vi "Create Init File.vi"(8 "error in (no error)":errorcluster caption="entrée d'erreur (pas d'erreur)", 9 "Nom du fichier ini":string, 10 "Répertoire de l'appli":path, 11 "UI Cam Basler in":refnum<class "UI Cam Basler.lvclass">) -> (0 "error out":errorcluster caption="sortie d'erreur", 3 "UI Cam Basler out":refnum<class "UI Cam Basler.lvclass">)   [LabVIEW 2023, in "UI Cam Basler.lvclass"]
uses:
  UI Cam Basler.lvclass
  UI Cam Basler.lvclass/UI Cam Basler.ctl
  83761873-ac89-497a-a2f6-ac3f21e5bc55.vi
  83761873-ac89-497a-a2f6-ac3f21e5bc55.vi/659df739-fa42-474c-bf03-f9ba45f35773.vi
  <vilib>/Utility/file.llb/Is Path and Not Empty.vi
  <vilib>/Utility/libraryn.llb/Librarian Path Location.vi
  <userlib>/_OpenG.lib/file/file.llb/File Exists__ogtk.vi
  <userlib>/_OpenG.lib/file/file.llb/File Exists - Scalar__ogtk.vi
  <userlib>/LV-TOML/lib/Parse TOML String.vi
  <userlib>/LV-TOML/lib/TOML to LabVIEW.vi
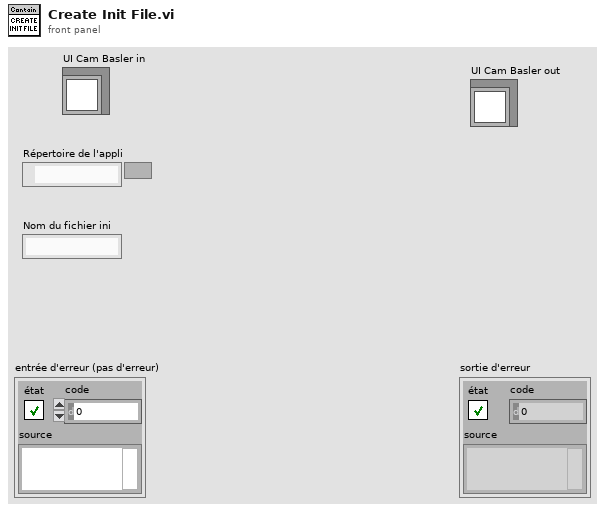
[diagram p1: front panel]
types:
  T1 = enum16{"open", "replace", "create", "open or create", "replace or create", "replace or create with confirmation"}
  T2 = typedef "UI Cam Basler.lvclass/Parsed Data Acquisition.ctl" = cluster{"Config Acquisition":cluster{"Camera name":string, "Gain":dbl, "Shutter(us)":dbl, "ROI":bool, "ROI coor":T3, "Palette":u32, "ModelName":string}}
  T3 = typedef "IMAQ Rectangle" = cluster{"Left":i32, "Top":i32, "Right":i32, "Bottom":i32, "Rotation":dbl}
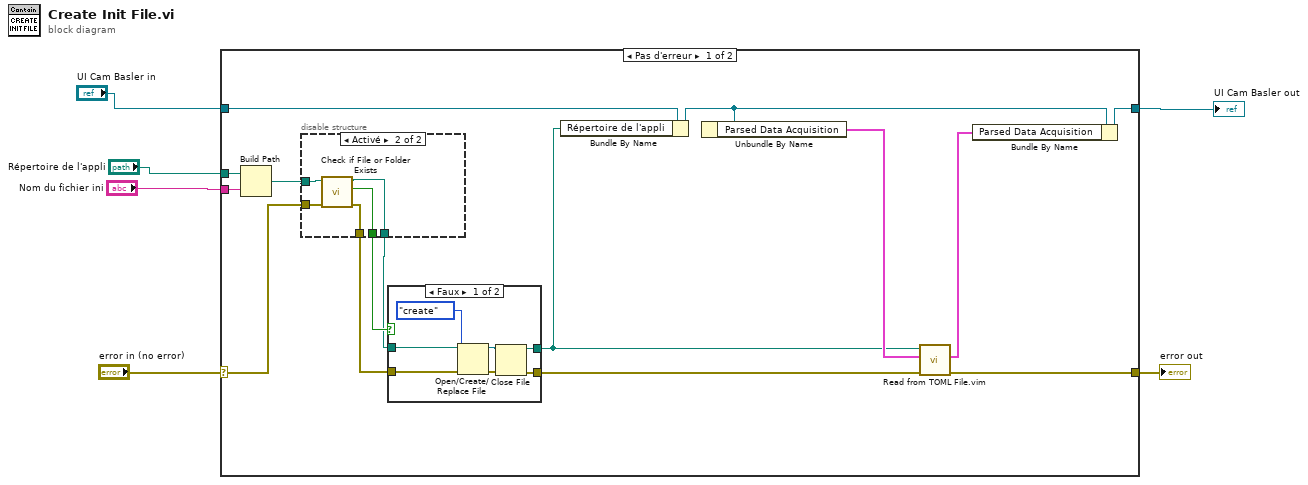
[diagram p0: block diagram]
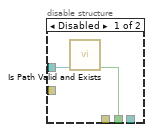
[diagram p2: hidden frame]
diagram:
  n1 = case shown="Pas d'erreur" "error in (no error)" {
    selector: "error in (no error)" -> [w9 w39]
    tunnel: [w15 w39] -> w5
    tunnel: [w11 w38] -> w1
    tunnel: "UI Cam Basler in" -> [w21 w38]
    tunnel: "Répertoire de l'appli" -> [w18 _]
    tunnel: "Nom du fichier ini" -> [w17 _]
    frame No Error {
      n2 = Build Path(base path=w18, name or relative path=w17) -> (appended path=w19:path)
      n3 = disable-structure shown="Activé" {
        disable-tunnel: [w23 w27] -> w20
        disable-tunnel: w19 -> [w22 w28]
        disable-tunnel: w9 -> [_ w26]
        disable-tunnel: [_ w25] -> w8
        disable-tunnel: [_ w24] -> w7
        frame Disabled {
          n4 = call <userlib>:"Is Path Valid and Exists.vi"("File/Folder Path"=w22) -> ("Valid and Exists?"=w23:bool)  [unwired: 9 in, 1 out]
        }
        frame Enabled {
          n5 = call <vilib>:"Check if File or Folder Exists.vi"("error in (no error)"=w26, "path"=w28) -> ("error out"=w25:errorcluster, "file or folder exists?"=w27:bool, "dup path"=w24:path)  [unwired: 7 in]
        }
      }
      n6 = case "Structure Condition" shown="Faux" w20 {
        tunnel: [w33 w37] -> w12
        tunnel: w7 -> [w35 w37]
        tunnel: w8 -> [w31 w36]
        tunnel: [w29 w36] -> w16
        frame False {
          n7 = Open/Create/Replace File(file path (use dialog)=w35, error in=w31, operation (0:open)=T1."create" ("opération (0 : open)")) -> (refnum out=w34:refnum<file>, error out=w30:errorcluster)  [unwired: 3 in, 1 out]
          n8 = Close File(refnum=w34, error in=w30) -> (path=w33:path, error out=w29:errorcluster)
        }
        frame True {
        }
      }
      n9 = Bundle By Name(cluster=w21, "Répertoire de l'appli"=w12) -> (w14:refnum<class "UI Cam Basler.lvclass">)
      n10 = Unbundle By Name(w14) -> ("Parsed Data Acquisition"=w13:T2)
      n11 = call "Read from TOML File.vim"("error in (no error)"=w16, "Default Value"=w13, "file path (use dialog)"=w12) -> ("error out"=w15:errorcluster, "Value"=w10:T2)  [unwired: 6 in, 1 out]
      n12 = Bundle By Name(cluster=w14, "Parsed Data Acquisition"=w10) -> (w11:refnum<class "UI Cam Basler.lvclass">)
    }
    frame Error {
    }
  }
  "error out" <- w5
  "UI Cam Basler out" <- w1
